vi "createReadAngleFrame.vi"(8 "error in (no error)":errorcluster, 11 "T7Inclinometer in":refnum<class "T7Inclinometer.lvclass">) -> (0 "error out":errorcluster, 2 "Message":u8[](array[numeric]), 3 "T7Inclinometer out":refnum<class "T7Inclinometer.lvclass">)   [LabVIEW 2016, in "RTT7Inclinometer.lvlib" / "T7Inclinometer.lvclass"]
uses:
  T7Inclinometer.lvclass
  Common_RT_Utilities/U8ArrayBuilderAutoIndexing/U8ArrayBuilderAutoIndexing.lvclass
  T7Inclinometer.lvclass/T7Inclinometer.ctl
  Common_RT_Utilities/CRC16/CRC16.lvclass
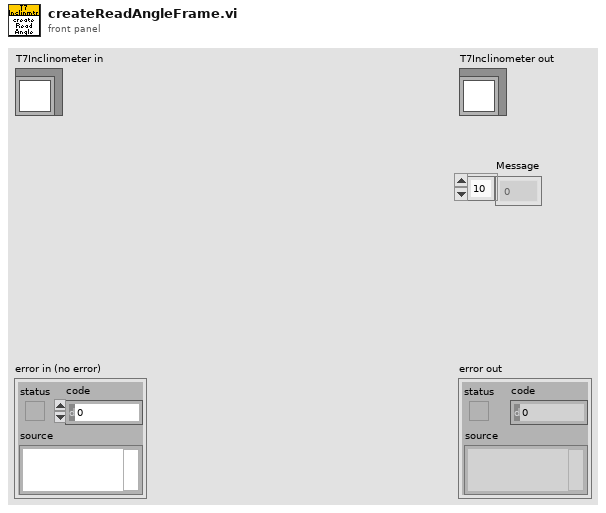
[diagram p1: front panel]
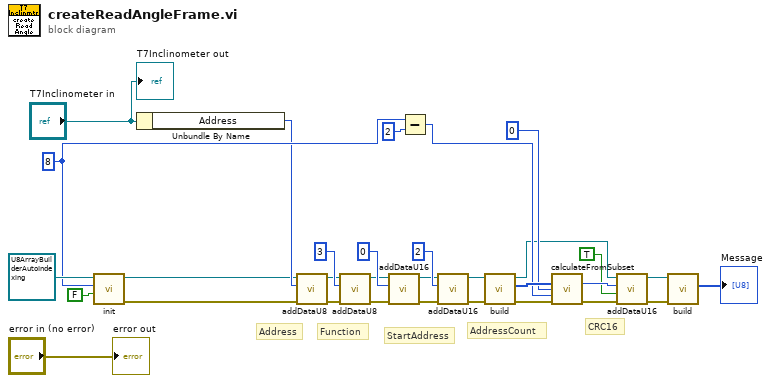
[diagram p0: block diagram]
diagram:
  w24 = 8 ("Size")
  # "CRC16"
  # "AddressCount"
  # "StartAddress"
  # "Function"
  # "Address"
  n1 = call "init.vi"("SwapBytes"=FALSE, "Size"=w24, "U8ArrayBuilderAutoIndexing in"=refnum<class "U8ArrayBuilderAutoIndexing.lvclass"> refnum ("RTUtilities.lvlib:U8ArrayBuilder.lvclass")) -> ("error out"=w1:errorcluster, "U8ArrayBuilderAutoIndexing out"=w2:refnum<class "U8ArrayBuilderAutoIndexing.lvclass">)  [unwired: 7 in]
  n2 = Unbundle By Name("T7Inclinometer in") -> ("Address"=w20:u8)
  n3 = call "addDataU8.vi"("error in (no error)"=w1, "Data"=w20, "U8ArrayBuilderAutoIndexing in"=w2) -> ("error out"=w17:errorcluster, "U8ArrayBuilderAutoIndexing out"=w18:refnum<class "U8ArrayBuilderAutoIndexing.lvclass">)  [unwired: 7 in]
  n4 = call "addDataU8.vi"("error in (no error)"=w17, "Data"=u8 3, "U8ArrayBuilderAutoIndexing in"=w18) -> ("error out"=w14:errorcluster, "U8ArrayBuilderAutoIndexing out"=w15:refnum<class "U8ArrayBuilderAutoIndexing.lvclass">)  [unwired: 7 in]
  n5 = call "addDataU16.vi"("error in (no error)"=w14, "Data"=u16 0, "U8ArrayBuilderAutoIndexing in"=w15) -> ("error out"=w11:errorcluster, "U8ArrayBuilderAutoIndexing out"=w12:refnum<class "U8ArrayBuilderAutoIndexing.lvclass">)  [unwired: 7 in]
  n6 = Subtract(x=w24, y=2) -> (x-y=w25:i32)
  n7 = call "addDataU16.vi"("error in (no error)"=w11, "Data"=u16 2, "U8ArrayBuilderAutoIndexing in"=w12) -> ("error out"=w8:errorcluster, "U8ArrayBuilderAutoIndexing out"=w9:refnum<class "U8ArrayBuilderAutoIndexing.lvclass">)  [unwired: 7 in]
  n8 = call "build.vi"("error in (no error)"=w8, "U8ArrayBuilderAutoIndexing in"=w9) -> ("error out"=w22:errorcluster, "Array"=w27:u8[], "U8ArrayBuilderAutoIndexing out"=w10:refnum<class "U8ArrayBuilderAutoIndexing.lvclass">)  [unwired: 7 in]
  n9 = call "calculateFromSubset.vi"("Data"=w27, "StartIndex"=0, "Length"=w25, "error in (no error)"=w22) -> ("CRC"=w6:u16, "error out"=w7:errorcluster)  [unwired: 9 in, 1 out]
  n10 = call "addDataU16.vi"("error in (no error)"=w7, "OverrideSwapBytes"=TRUE, "Data"=w6, "U8ArrayBuilderAutoIndexing in"=w10) -> ("error out"=w4:errorcluster, "U8ArrayBuilderAutoIndexing out"=w3:refnum<class "U8ArrayBuilderAutoIndexing.lvclass">)  [unwired: 6 in]
  n11 = call "build.vi"("error in (no error)"=w4, "U8ArrayBuilderAutoIndexing in"=w3) -> ("Array"=→"Message":u8[])  [unwired: 7 in, 2 out]
  "error out" <- "error in (no error)"
  "T7Inclinometer out" <- "T7Inclinometer in"
